vi "PH_Cam_BaseClass.request Cam Settings.vi"(2 "Cam Instance":string, 5 "error in (no error)":errorcluster) -> (15 "Cam Setting Information":string="N/A", 16 "Error getting the Data?":bool, 17 "Cam Settings":T1={"Cam ID"="N/A", "Gain"=nan, "Brightness"=nan, "Shutter"=nan, "Mode"=-1}, 19 "error out":errorcluster)   [LabVIEW 2014, in "PH_Cam_BaseClass.lvlib"]
doc: "By this VI the current camera settings published via a DIM service are read."
uses:
  PH_Cam_BaseClass.lvlib
  PH_Cam_BaseClass.Settings.ctl
  lib.lib/DimLVEvent/LVDimInterface/LVDimInterface.lvlib
  CSCore/CSSystem/CoreLib/CoreLib.lvlib
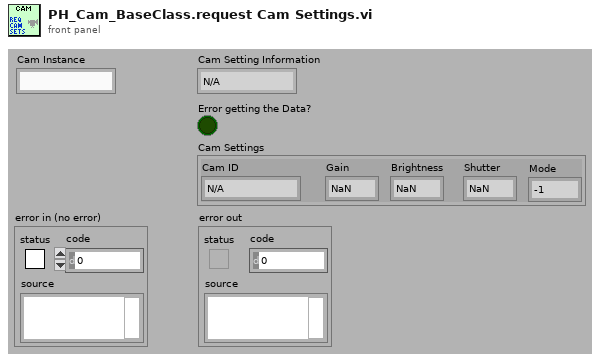
[diagram p1: front panel]
types:
  T1 = typedef "PH_Cam_BaseClass.lvlib/PH_Cam_BaseClass.Settings.ctl" = cluster{"Cam ID":string, "Gain":dbl, "Brightness":dbl, "Shutter":dbl, "Mode":i32}
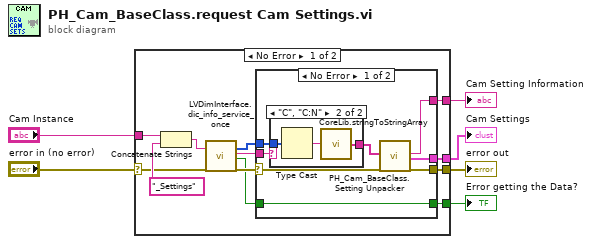
[diagram p0: block diagram]
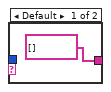
[diagram p2: hidden frame]
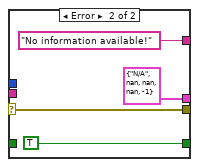
[diagram p3: hidden frame]
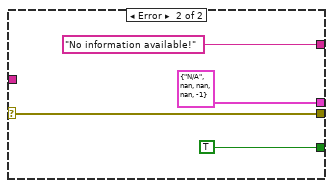
[diagram p4: hidden frame]
diagram:
  n1 = case shown="No Error" "error in (no error)" {
    selector: "error in (no error)" -> [w8 w37]
    tunnel: "Cam Instance" -> [w18 _]
    tunnel: [w13 T1 {"Cam ID"="N/A", "Gain"=nan, "Brightness"=nan, "Shutter"=nan, "Mode"=-1} ("Cam Settings")] -> w5
    tunnel: [w11 w37] -> w4
    tunnel: [w9 TRUE ("timed out?")] -> w3
    tunnel: [w7 "No information available!" ("Cam Setting Information")] -> w1
    frame No Error {
      n2 = Concatenate Strings(w18, "_Settings" ("string")) -> (w16:string)
      n3 = call "LVDimInterface.dic_info_service_once.vi"("serviceName"=w16, "error in (no error)"=w8) -> ("data"=w14:i8[], "typeDescriptor"=w15:string, "timed out?"=w10:bool, "error out"=w12:errorcluster)  [unwired: 14 in]
      n4 = case shown="No Error" w12 {
        selector: w12 -> [w23 w34]
        tunnel: [w22 w34] -> w11
        tunnel: w15 -> [w26 _]
        tunnel: w14 -> [w25 _]
        tunnel: [w21 T1 {"Cam ID"="N/A", "Gain"=nan, "Brightness"=nan, "Shutter"=nan, "Mode"=-1} ("Cam Settings")] -> w13
        tunnel: w10 -> [w20 _]
        tunnel: [w20 TRUE ("timed out?")] -> w9
        tunnel: [w19 "No information available!" ("Cam Setting Information")] -> w7
        frame No Error {
          n5 = case shown="\"C\", \"C:N\"" w26 {
            tunnel: w25 -> [_ w30]
            tunnel: [string[] [] ("Array") w28] -> w24
            frame Default {
            }
            frame "C", "C:N" {
              n6 = Type Cast(x=w30) -> (*(type *) &x=w29:string)  [unwired: 1 in]
              n7 = call "CoreLib.stringToStringArray.vi"("String"=w29) -> ("Array"=w28:string[])
            }
          }
          n8 = call "PH_Cam_BaseClass.Setting Unpacker.vi"("Cam Settings Array"=w24, "error in (no error)"=w23) -> ("Cam Setting Information"=w19:string, "Cam Settings"=w21:T1, "error out"=w22:errorcluster)  [unwired: 15 in]
        }
        frame Error {
        }
      }
    }
    frame Error {
    }
  }
  "Error getting the Data?" <- w3
  "error out" <- w4
  "Cam Settings" <- w5
  "Cam Setting Information" <- w1
